vi "Get DataRow (String).vi"(8 "error in (no error)":errorcluster, 10 "index":i32, 11 "DataTable in":refnum<class "DataTable.lvclass">) -> (0 "error out":errorcluster, 2 "Array":string[](array[string]), 3 "DataTable out":refnum<class "DataTable.lvclass">)   [LabVIEW 2016, in "DataGrid.lvlib" / "DataTable.lvclass"]
uses:
  <userlib>/LabVIEWdotNetDataGrid/source/DataTable/DataTable.lvclass
  <userlib>/LabVIEWdotNetDataGrid/source/DataTable/DataTable.lvclass/DataTable.ctl
  System.Data
  <userlib>/LabVIEWdotNetDataGrid/source/GridColumn/GridColumn.lvclass/GridColumn.ctl
  <userlib>/LabVIEWdotNetDataGrid/source/GridColumn/Read datatype.vi
  <vilib>/Utility/error.llb/Error Cluster From Error Code.vi
  <vilib>/ErrorRing/Error Ring.xnode
  <userlib>/LabVIEWdotNetDataGrid/source/GridColumn/GridColumn.lvclass
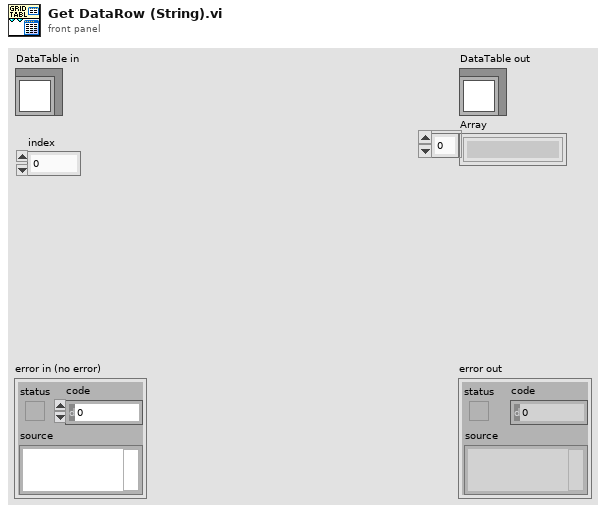
[diagram p1: front panel]
types:
  T1 = typedef "DataGrid.lvlib/GridColumn.lvclass/ColumnType.ctl" = enum16{"string", "image", "check", "numeric", "timestamp", "button", "combo", "link"}
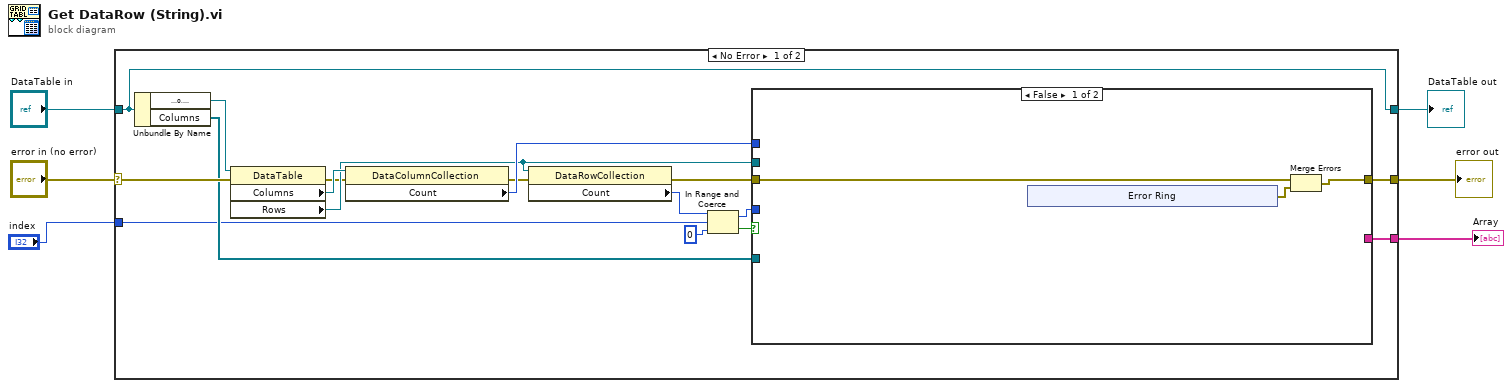
[diagram p0: block diagram]
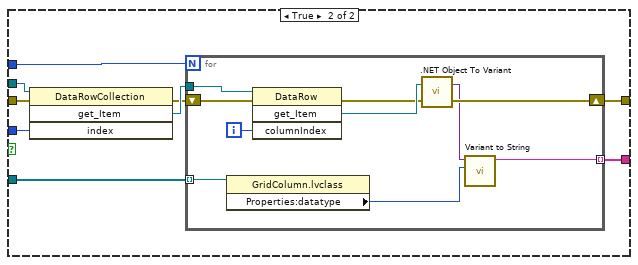
[diagram p2: hidden frame]
diagram:
  n1 = case shown="No Error" "error in (no error)" {
    selector: "error in (no error)" -> [w17 w50]
    tunnel: [w16 w50] -> w5
    tunnel: [w23 w51] -> w3
    tunnel: "DataTable in" -> [w23 w51]
    tunnel: [w12 _] -> w2
    tunnel: "index" -> [w7 _]
    frame No Error {
      n2 = Unbundle By Name(w23) -> ("DataTable"=w22:refnum<k24>, "Columns"=w13:refnum<class "GridColumn.lvclass">[])
      n3 = property class="DataTable"(reference=w22, error in=w17) -> (error out=w18:errorcluster, "Columns"=w21:refnum<k24>, "Rows"=w19:refnum<k24>)  [unwired: 1 out]
      n4 = property class="DataColumnCollection"(reference=w21, error in=w18) -> (error out=w15:errorcluster, "Count"=w20:i32)  [unwired: 1 out]
      n5 = property class="DataRowCollection"(reference=w19, error in=w15) -> (error out=w14:errorcluster, "Count"=w10:i32)  [unwired: 1 out]
      n6 = In Range and Coerce(upper limit=w10, x=w7, lower limit=0 ("x")) -> (coerced(x)=w11:i32, In Range?=w8:bool)
      n7 = case shown="False" w8 {
        tunnel: w20 -> [_ w39]
        tunnel: w19 -> [_ w38]
        tunnel: [w25 w37] -> w16
        tunnel: w14 -> [w26 w36]
        tunnel: w13 -> [_ w35]
        tunnel: [_ w34] -> w12
        tunnel: w11 -> [_ w31]
        frame False {
          n8 = xnode "Error Ring"() -> ("error out"=w24:errorcluster)
          n9 = Merge Errors(w26, w24) -> (w25:errorcluster)
        }
        frame True {
          n10 = invoke class="DataRowCollection" method="get_Item"(reference=w38, error in=w36, "index"=w31) -> (error out=w32:errorcluster, "get_Item"=w33:refnum<k24>)  [unwired: 1 in, 2 out]
          n11 = for {
            N: w39 -> [_]
            tunnel: w33 -> [w49]
            shift-right: [w44] -> w37
            shift-left: w32 -> [w47]
            tunnel: w35 -> [w43] mode=indexing
            tunnel: [w40] -> w34 mode=indexing
            i -> [w48]
            n12 = property class="GridColumn.lvclass"(reference=w43) -> ("Properties:datatype"=w42:T1)  [unwired: 1 in, 2 out]
            n13 = invoke class="DataRow" method="get_Item"(reference=w49, error in=w47, "columnIndex"=w48) -> (error out=w45:errorcluster, "get_Item"=w46:refnum<k24>)  [unwired: 1 in, 2 out]
            n14 = call <vilib>:".NET Object To Variant.vi"("error in (no error)"=w45, ".NET object"=w46) -> ("error out"=w44:errorcluster, "variant"=w41:variant)
            n15 = call <userlib>:"Variant to String.vi"("datatype"=w42, "Variant"=w41) -> ("String"=w40:string)  [unwired: 8 in, 1 out]
          }
        }
      }
    }
    frame Error {
    }
  }
  "error out" <- w5
  "DataTable out" <- w3
  "Array" <- w2
